vi "Test_InsertItems.vi"(8 "error in (no error)":errorcluster, 11 "TestCase in":refnum<class "ListImp_Functional.lvclass">) -> (0 "error out":errorcluster, 3 "TestCase out":refnum<class "ListImp_Functional.lvclass">)   [LabVIEW 2009, in "ListImp_Functional.lvclass"]
uses:
  ListImp_Functional.lvclass
  ListImp_Functional.lvclass/ListImp_Functional.ctl
  source/Lists/List/List.lvclass
  source/Lists.Interfaces/String/String.lvclass
  UnitTestComparisons/UnitTestComparisons.lvlib
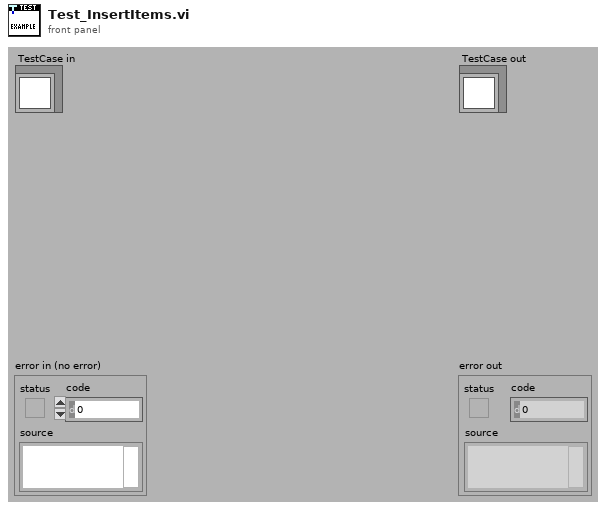
[diagram p1: front panel]
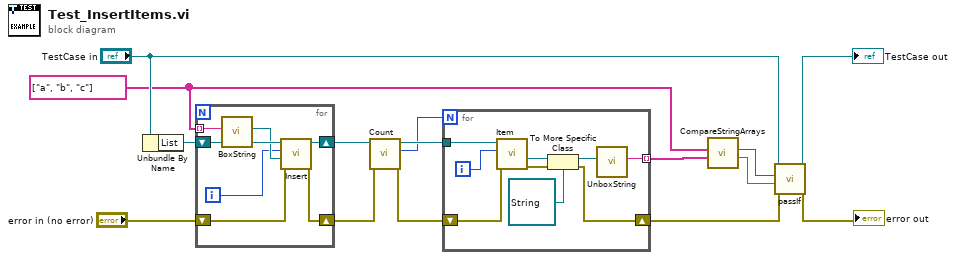
[diagram p0: block diagram]
diagram:
  w3 = string[] ["a", "b", "c"]
  n1 = Unbundle By Name("TestCase in") -> ("List"=w12:refnum<class "List.lvclass">)
  n2 = for {
    tunnel: w3 -> [w19] mode=indexing
    shift-right: [w21] -> w9
    shift-left: w12 -> [w22]
    shift-right: [w16] -> w7
    shift-left: "error in (no error)" -> [w17]
    i -> [w18]
    n3 = call "BoxString.vi"("String"=w19) -> ("String out"=w20:refnum<class "String.lvclass">)  [unwired: 10 in]
    n4 = call-dynamic "Insert.vi"("error in (no error)"=w17, "Item"=w20, "Index"=w18, "List in"=w22) -> ("error out"=w16:errorcluster, "List out"=w21:refnum<class "List.lvclass">)  [unwired: 6 in]
  }
  n5 = call-dynamic "Count.vi"("error in (no error)"=w7, "List in"=w9) -> ("error out"=w6:errorcluster, "Number of Items"=w5:i32, "List out"=w8:refnum<class "List.lvclass">)  [unwired: 7 in]
  n6 = for {
    N: w5 -> [_]
    tunnel: w8 -> [w31]
    shift-right: [w25] -> w10
    shift-left: w6 -> [w30]
    tunnel: [w23] -> w4 mode=indexing
    i -> [w29]
    n7 = call-dynamic "Item.vi"("error in (no error)"=w30, "Index"=w29, "List in"=w31) -> ("error out"=w26:errorcluster, "Item"=w28:refnum<class>)  [unwired: 6 in, 1 out]
    n8 = To More Specific Class(target class=refnum<class "String.lvclass"> refnum ("LapDog.Collections.v0.Lists.Interfaces.lvlib:String.lvclass"), reference=w28, error in=w26) -> (specific class reference=w27:refnum<class "String.lvclass">, error out=w25:errorcluster)
    n9 = call "UnboxString.vi"("String in"=w27) -> ("String"=w23:string)  [unwired: 10 in]
  }
  n10 = call "CompareStringArrays.vi"("Expected Strings"=w4, "Actual Strings"=w3) -> ("Message"=w1:string, "Equal?"=w2:bool)  [unwired: 8 in]
  n11 = call-dynamic "passIf.vi"("error in (no error)"=w10, "message (\"\")"=w1, "pass"=w2, "TestCase in"="TestCase in") -> ("error out"=→"error out":errorcluster, "TestCase out"=→"TestCase out":refnum<class "ListImp_Functional.lvclass">)  [unwired: 6 in]
